vi "Configure Conversion Loss Table.vi"(8 "error in (no error)":errorcluster {"code" format="%.0x"}, 9 "conversion loss":dbl[](array[numeric])=[0.0] format="%^.2e", 10 "frequency":dbl[](array[numeric])=[0.0] caption="frequency (Hz)" format="%^.2e", 11 "instrument handle":refnum<k15>) -> (0 "error out":errorcluster {"code" format="%.0x"}, 3 "instrument handle out":refnum<k15>)   [LabVIEW 2009, in "Keysight XSAn.lvlib"]
doc: "This VI configures the conversion loss table by specifying a frequency and a power loss pair.\n\nSupported Models: M9290A, N8973B, N8974B, N8975B, N8976B, N9000A, N9000B, N9010A, N9010B, N9020A, N9020B, N9030A, N9030B, N9038A, N9040B, N9041B, SPN9003A, SPN9026A"
uses:
  <instrlib>/Keysight XSAn/Keysight XSAn.lvlib
  AgXSAn.dll
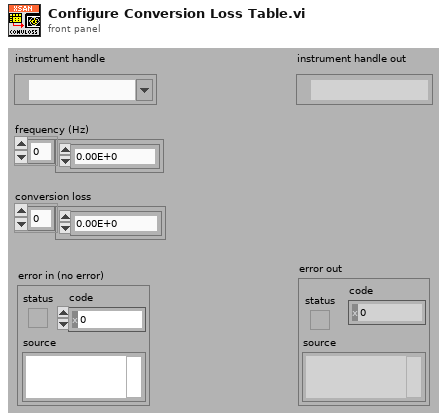
[diagram p1: front panel]
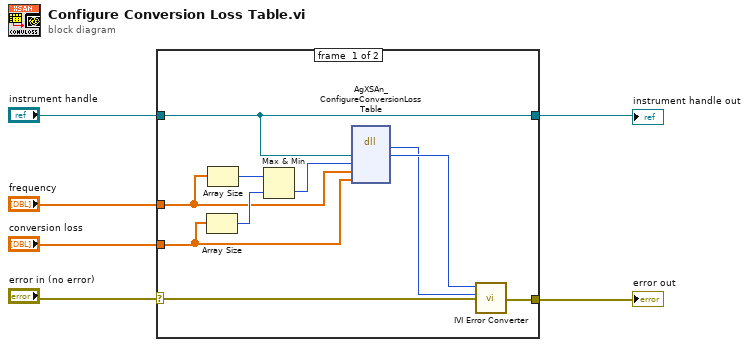
[diagram p0: block diagram]
diagram:
  n1 = case shown="No Error" "error in (no error)" {
    selector: "error in (no error)" -> [w14 w18]
    tunnel: [w15 w18] -> w5
    tunnel: "instrument handle" -> [w7 w17]
    tunnel: "frequency" -> [w9 _]
    tunnel: "conversion loss" -> [w8 _]
    tunnel: [w7 w17] -> w1
    frame #0 {
      n2 = Array Size(array=w8) -> (size(s)=w11:i32)
      n3 = Array Size(array=w9) -> (size(s)=w12:i32)
      n4 = Max & Min(x=w12, y=w11) -> (min(x,y)=w10:i32)  [unwired: 1 out]
      n5 = dll-call lib="AgXSAn**.dll" fn="AgXSAn_ConfigureConversionLossTable" ("LabVIEW:IviSpecAn_ConfigureConversionLossTable")("instrument handle"=w7, "count"=w10, "frequency"=w9, "conversion loss"=w8) -> ("Status"=w13:i32, "instrument handle"=w16:u32)  [unwired: 6 in, 2 out]
      n6 = call <instrlib>:"IVI Error Converter.vi"("error in (no error)"=w14, "IVI error code (0)"=w13, "instrument handle"=w16) -> ("error out"=w15:errorcluster)  [unwired: 7 in, 1 out]
    }
    frame #1 {
    }
  }
  "error out" <- w5
  "instrument handle out" <- w1
